vi "hdt_ort_averageChannels.vi"(8 "outSteamSelect":u8(ring) items=["PID/ORT", "SICM"], 11 "enableOutput":bool) -> ()   [LabVIEW 2016]
uses:
  <vilib>/rvi/DataTransferAndStorage/Container/XNode/niFpgaContainer.xnode
  <vilib>/rvi/FIFO/Fifo_Resource/nirvififoEmulationRead.vi
  <vilib>/eio/EIONode/EIONode.xnode
  <instrlib>/_niInstr/Basic Elements/v1/FPGA/niInstr Basic Elements v1 FPGA.lvlib
  <vilib>/rvi/FXPMathLib/FxpInterpret/XNode/nifxpmath_Interpret.xnode
  <vilib>/rvi/FIFO/Fifo_Resource/nirvififoEmulationWrite.vi
  <vilib>/rvi/DataTransferAndStorage/Register/Emulation/niFpgaRegisterEmulation.vi
  <vilib>/rvi/eio/common/nirviEmuTemplateMethod_errors.vi
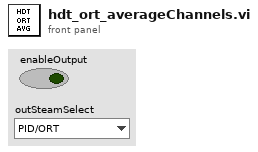
[diagram p1: front panel]
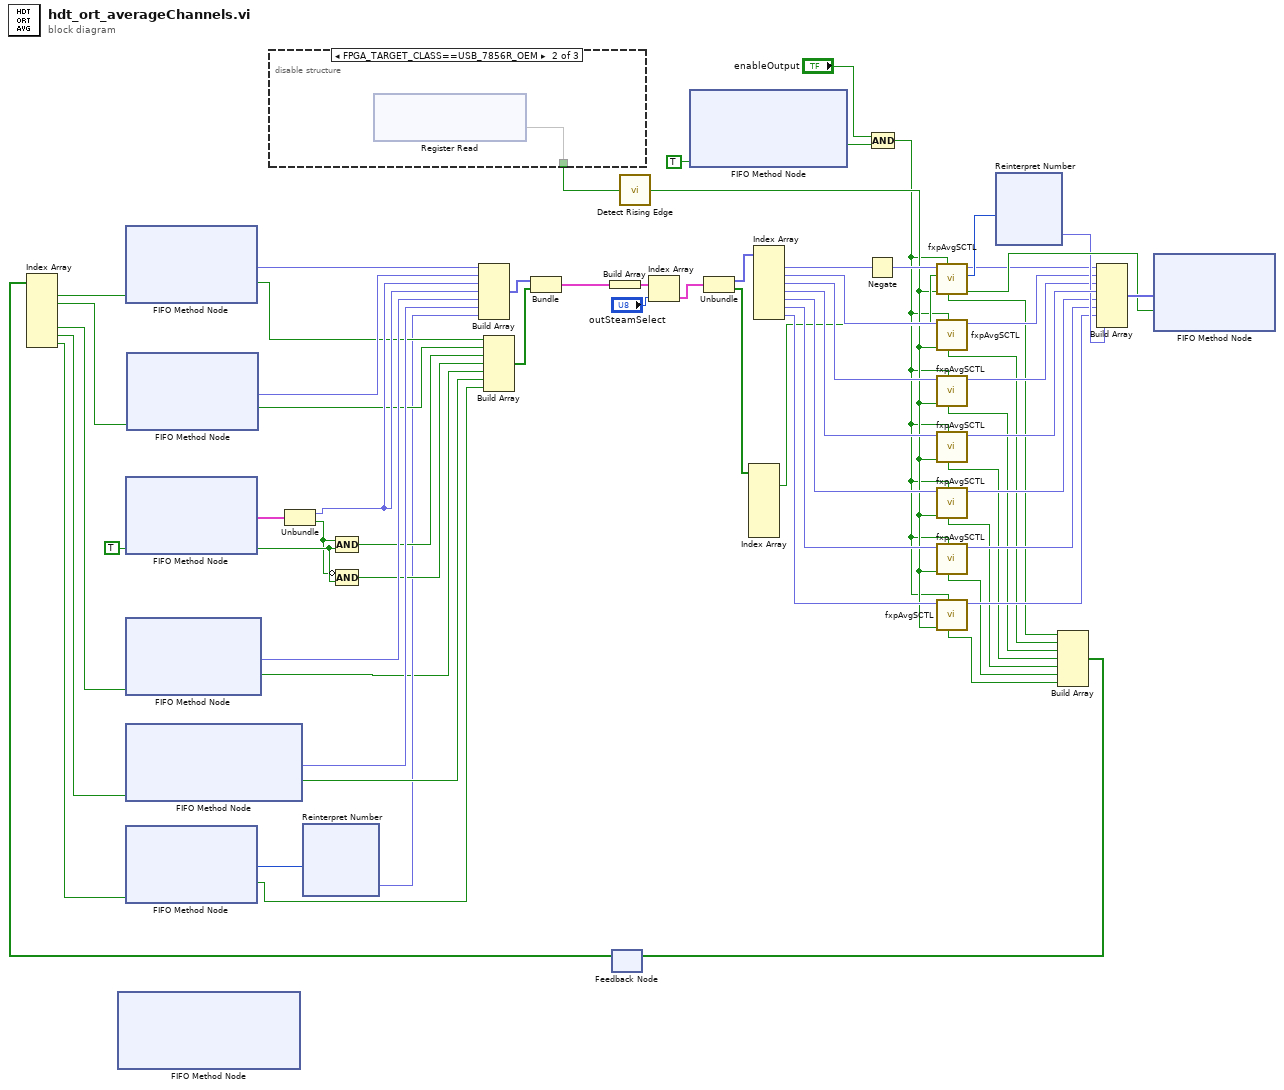
[diagram p0: block diagram]
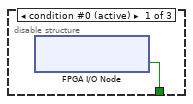
[diagram p2: hidden frame]
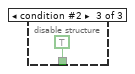
[diagram p3: hidden frame]
diagram:
  n1 = xnode ("FIFO Method Node")() -> ()  [unwired: 2 in, 3 out]
  n2 = xnode ("FIFO Method Node")("Ready for Output"=TRUE) -> ("Element"=w49:cluster{"slope":fxp<+/-,22,1>, "forward":bool}, "Output Valid"=w60:bool)  [unwired: 1 in, 1 out]
  n3 = disable-structure shown="FPGA_TARGET_CLASS==USB_7856R_OEM" {
    disable-tunnel: [w67 w68 TRUE ("outputEnable")] -> w48
    frame condition #0 (active) {
      n4 = xnode "FPGA I/O Node"() -> ("outputEnable"=w67:bool)  [unwired: 1 in, 1 out]
    }
    frame condition #1 {
      n5 = xnode ("Register Read")() -> ("Data"=w68)  [unwired: 1 in, 1 out]
    }
    frame condition #2 {
    }
  }
  n6 = Unbundle(w49) -> ("slope"=w44:fxp<+/-,22,1>, "forward"=w58:bool)
  n7 = Compound Arithmetic op=AND(w58, w60) -> (w39:bool)
  n8 = Compound Arithmetic op=AND(invert w58, w60) -> (w38:bool)
  n9 = feedback #1() -> (w11:bool[])  [unwired: 1 in]
  n10 = Index Array(array=w11) -> (element #1=w8:bool, element #2=w7:bool, element #5=w4:bool, element #6=w5:bool, element #7=w6:bool)  [unwired: 7 in, 2 out]
  n11 = xnode ("FIFO Method Node")("Ready for Output"=w8) -> ("Element"=w28:fxp<+/-,22,1>, "Output Valid"=w41:bool)  [unwired: 1 in, 1 out]
  n12 = xnode ("FIFO Method Node")("Ready for Output"=w4) -> ("Element"=w43:fxp<+/-,22,1>, "Output Valid"=w10:bool)  [unwired: 1 in, 1 out]
  n13 = xnode ("FIFO Method Node")("Ready for Output"=w5) -> ("Element"=w42:fxp<+/-,18,1>, "Output Valid"=w37:bool)  [unwired: 1 in, 1 out]
  n14 = xnode ("FIFO Method Node")("Ready for Output"=w6) -> ("Element"=w46:i16, "Output Valid"=w9:bool)  [unwired: 1 in, 1 out]
  n15 = xnode ("FIFO Method Node")("Ready for Output"=w7) -> ("Element"=w45:fxp<+/-,22,1>, "Output Valid"=w40:bool)  [unwired: 1 in, 1 out]
  n16 = xnode "Reinterpret Number"("x"=w46) -> ("y"=w21:fxp<+/-,16,1>)
  n17 = Build Array(w28, w45, w44, w44, w43, w42, w21) -> (w36:fxp<+/-,22,1>[])
  n18 = Build Array(w41, w40, w39, w38, w10, w37, w9) -> (w35:bool[])
  n19 = Bundle(w36, w35) -> (w34:cluster{fxp<+/-,22,1>[], bool[]})  [unwired: 1 in]
  n20 = Build Array(w34) -> (w33:cluster{fxp<+/-,22,1>[], bool[]}[])
  n21 = call <instrlib>:"Detect Rising Edge.vi"("signal"=w48) -> ("edge detected"=w2:bool)  [unwired: 14 in]
  n22 = Index Array(array=w33, index="outSteamSelect") -> (element=w31:cluster{fxp<+/-,22,1>[], bool[]})
  n23 = xnode ("FIFO Method Node")("Ready for Output"=TRUE) -> ("Output Valid"=w64:bool)  [unwired: 1 in, 2 out]
  n24 = Unbundle(w31) -> (w30:fxp<+/-,22,1>[], w29:bool[])
  n25 = Index Array(array=w29) -> (element #1=w3:bool)  [unwired: 7 in, 6 out]
  n26 = Index Array(array=w30) -> (element #1=w27:fxp<+/-,22,1>, element #2=w26:fxp<+/-,22,1>, element #3=w25:fxp<+/-,22,1>, element #4=w24:fxp<+/-,22,1>, element #5=w23:fxp<+/-,22,1>, element #6=w22:fxp<+/-,22,1>, element #7=w20:fxp<+/-,22,1>)  [unwired: 7 in]
  n27 = Negate(x=w27) -> (-x=w66:fxp<+/-,23,2>)
  n28 = Compound Arithmetic op=AND("enableOutput", w64) -> (w1:bool)
  n29 = call "fxpAvgSCTL.vi"("reset"=w1, "clear"=w2, "inputValid"=w3, "input"=w66) -> ("outputValid"=w62:bool, "noAvg"=w56:u16, "average"=w50:fxp<+/-,22,1>, "readyForInput"=w19:bool)  [unwired: 4 in]
  n30 = call "fxpAvgSCTL.vi"("reset"=w1, "clear"=w2, "input"=w26) -> ("average"=w51:fxp<+/-,22,1>, "readyForInput"=w18:bool)  [unwired: 5 in, 2 out]
  n31 = call "fxpAvgSCTL.vi"("reset"=w1, "clear"=w2, "input"=w25) -> ("average"=w52:fxp<+/-,22,1>, "readyForInput"=w17:bool)  [unwired: 5 in, 2 out]
  n32 = call "fxpAvgSCTL.vi"("reset"=w1, "clear"=w2, "input"=w24) -> ("average"=w59:fxp<+/-,22,1>, "readyForInput"=w16:bool)  [unwired: 5 in, 2 out]
  n33 = call "fxpAvgSCTL.vi"("reset"=w1, "clear"=w2, "input"=w23) -> ("average"=w53:fxp<+/-,22,1>, "readyForInput"=w15:bool)  [unwired: 5 in, 2 out]
  n34 = call "fxpAvgSCTL.vi"("reset"=w1, "clear"=w2, "input"=w22) -> ("average"=w54:fxp<+/-,22,1>, "readyForInput"=w14:bool)  [unwired: 5 in, 2 out]
  n35 = call "fxpAvgSCTL.vi"("reset"=w1, "clear"=w2, "input"=w20) -> ("average"=w55:fxp<+/-,22,1>, "readyForInput"=w13:bool)  [unwired: 5 in, 2 out]
  n36 = xnode "Reinterpret Number"("x"=w56) -> ("y"=w57:fxp<+,16,1>)
  n37 = Build Array(w19, w18, w17, w16, w15, w14, w13) -> (w12:bool[])
  n38 = feedback-in #1(w12) -> ()
  n39 = Build Array(w50, w51, w52, w59, w53, w54, w55, w57) -> (w65:fxp<+/-,23,2>[])
  n40 = xnode ("FIFO Method Node")("Element"=w65, "Input Valid"=w62) -> ()  [unwired: 1 in, 2 out]
